vi "Merge_row_DBL_values.vi"(2 "Present Row values":dbl[](array[numeric]) format="%.2f", 3 "Present Channels":string[](array[string]), 4 "Desired Channels":string[](array[string])) -> (0 "Merged?":bool, 1 "Desired Row values":dbl[](array[numeric]) format="%.2f")   [LabVIEW 2010]
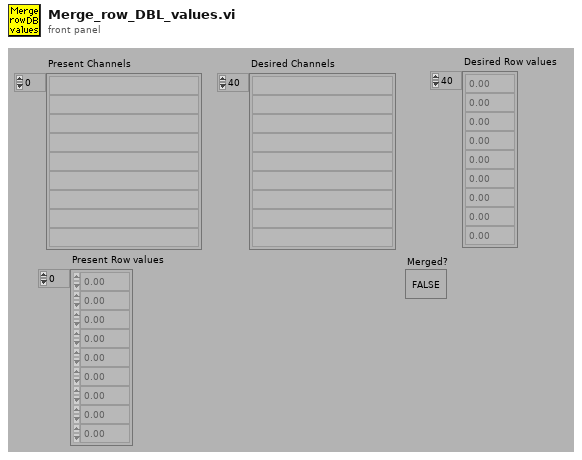
[diagram p1: front panel]
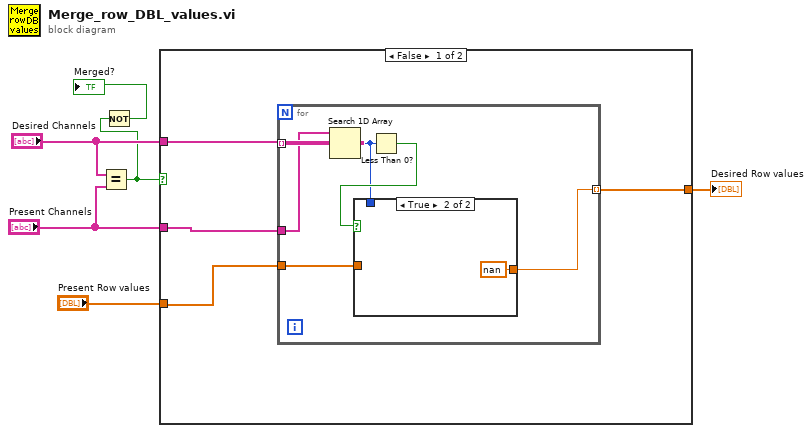
[diagram p0: block diagram]
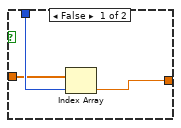
[diagram p2: hidden frame]
diagram:
  n1 = Equal?(x="Desired Channels", y="Present Channels") -> (x = y?=w2:bool)
  n2 = Not(x=w2) -> (.not. x?=→"Merged?":bool)
  n3 = case shown="False" w2 {
    tunnel: "Present Channels" -> [w10 _]
    tunnel: "Desired Channels" -> [w9 _]
    tunnel: [w8 w21] -> w4
    tunnel: "Present Row values" -> [w7 w21]
    frame False {
      n4 = for {
        tunnel: w10 -> [w16]
        tunnel: w9 -> [w15] mode=indexing
        tunnel: w7 -> [w12]
        tunnel: [w11] -> w8 mode=indexing
        n5 = Search 1D Array(1D array=w16, element=w15) -> (index of element=w13:i32)  [unwired: 1 out]
        n6 = Less Than 0?(x=w13) -> (x < 0?=w14:bool)
        n7 = case shown="True" w14 {
          tunnel: w13 -> [w19 _]
          tunnel: w12 -> [w18 _]
          tunnel: [w17 nan] -> w11
          frame False {
            n8 = Index Array(array=w18, index=w19) -> (element=w17:dbl)
          }
          frame True {
          }
        }
      }
    }
    frame True {
    }
  }
  "Desired Row values" <- w4
